vi "Piston Control.vi"   [LabVIEW 2019]
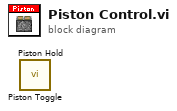
[diagram p0: block diagram]
diagram:
  n1 = call "Piston Toggle.vi"() -> ()  [unwired: 2 in, 1 out]
  n2 = call "Piston Hold.vi"() -> ()  [unwired: 2 in, 1 out]
